vi "Read Multi Value as String.vi"(8 "error in (no error)":errorcluster, 10 "Tag":string[](array[string]), 11 "Var Bus in":refnum<class "Omni_Bus.lvclass">) -> (0 "error out":errorcluster, 2 "String":string[](array[string]), 3 "Var Bus out":refnum<class "Omni_Bus.lvclass">)   [LabVIEW 2021, in "Omni_Bus.lvclass"]
uses:
  Omni_Bus.lvclass
  <vilib>/TSA/Abstract Data Classes/Abs_Types/Value/Abs_Value.lvclass
  Omni_Bus.lvclass/Omni_Bus.ctl
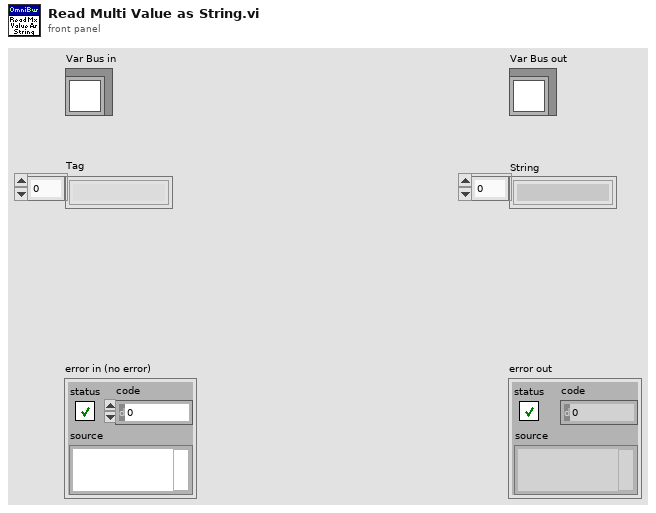
[diagram p1: front panel]
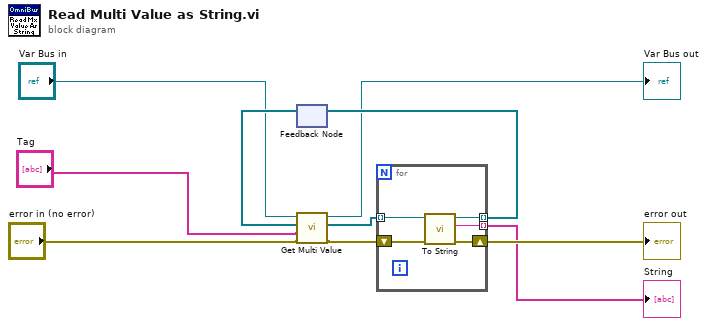
[diagram p0: block diagram]
diagram:
  n1 = feedback #1() -> (w3:refnum<class "Abs_Value.lvclass">[])  [unwired: 1 in]
  n2 = call-dynamic "Get Multi Value.vi"("error in (no error)"="error in (no error)", "Tag"="Tag", "Value Type"=w3, "Var Bus in"="Var Bus in") -> ("error out"=w7:errorcluster, "Value Out"=w6:refnum<class "Abs_Value.lvclass">[], "Var Bus out"=→"Var Bus out":refnum<class "Omni_Bus.lvclass">)  [unwired: 5 in]
  n3 = for {
    tunnel: [w14] -> w9 mode=indexing
    tunnel: [w13] -> w8 mode=indexing
    tunnel: w6 -> [w11] mode=indexing
    shift-right: [w15] -> w10
    shift-left: w7 -> [w12]
    n4 = call-dynamic "To String.vi"("error in (no error)"=w12, "Types in"=w11) -> ("error out"=w15:errorcluster, "String"=w14:string, "Types out"=w13:refnum<class "Abs_Value.lvclass">)  [unwired: 7 in]
  }
  "error out" <- w10
  "String" <- w9
  n5 = feedback-in #1(w8) -> ()
